vi "Acquire Spectrum.vi"(4 "Acquisition Time (s)":dbl=0.001 format="%.2p", 5 "Span (Hz)":dbl=192000.0 format="%.3p", 6 "Sample Rate (S/s)":dbl=50000000.0 format="%.2p", 7 "Reference Level":dbl format="%.2f", 8 "error in (no error)":errorcluster, 9 "RBW (Hz)":dbl=10000.0 format="%.3p", 10 "Center Frequency (Hz)":dbl=1000000000.0 format="%.6p", 11 "Instrument Handle In":refnum<k21>) -> (0 "error out":errorcluster, 2 "Spectrum":cluster{"x0":dbl, "dx":dbl, "y":sgl[]}(graph), 3 "Instrument Handle Out":refnum<k21>)   [LabVIEW 2018]
uses:
  <vilib>/RFmx/SpecAn/mx/RFmxSpecAn.llb/RFmxSpecAn Select Measurement (Single).vi
  <vilib>/RFmx/SpecAn/mx/RFmxSpecAn.llb/RFmxSpecAn Spectrum Fetch Spectrum.vi
  <vilib>/RFmx/SpecAn/mx/RFmxSpecAn.llb/RFmxSpecAn Configure IQ Power Edge Trigger.vi
panel:
  in  "Frequency Reference Source":string(combo)="OnboardClock"
  in  "Frequency (Hz)":dbl=10000000.0 format="%.6p"
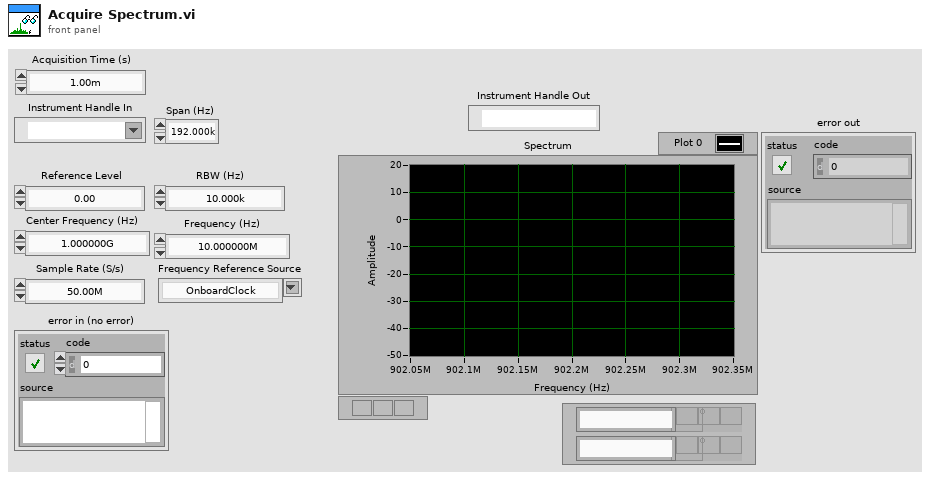
[diagram p1: front panel]
types:
  T1 = enum16{"ACP", "CCDF", "CHP", "FCnt", "Harmonics", "OBW", "SEM", "Spectrum", "Spur", "TXP", "AMPM", "DPD", "IQ", "IM", "NF", "PhaseNoise", "PAVT"}
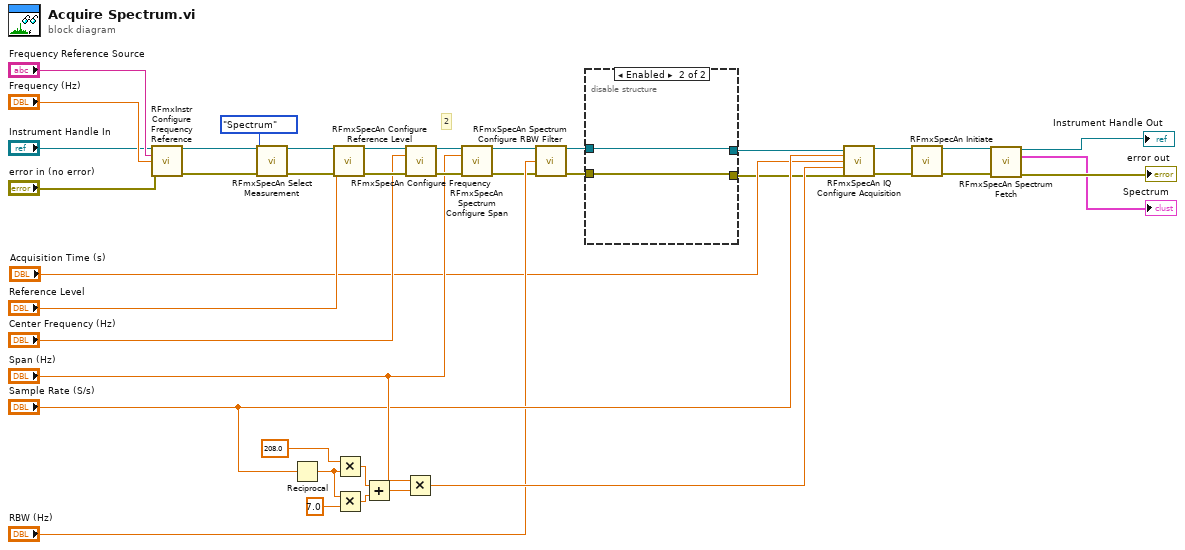
[diagram p0: block diagram]
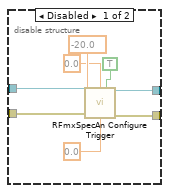
[diagram p2: hidden frame]
diagram:
  # "2"
  n1 = call <vilib>:"RFmxInstr Configure Frequency Reference.vi"("Instrument Handle In"="Instrument Handle In", "Frequency Reference Source"="Frequency Reference Source", "Frequency (Hz)"="Frequency (Hz)", "error in (no error)"="error in (no error)") -> ("Instrument Handle Out"=w16:refnum<k21>, "error out"=w15:errorcluster)  [unwired: 10 in]
  n2 = call-poly <vilib>:"RFmxSpecAn Select Measurement.vi"("Instrument Handle In"=w16, "Measurement"=T1."Spectrum", "error in (no error)"=w15) -> ("Instrument Handle Out"=w18:refnum<k21>, "error out"=w17:errorcluster)  [unwired: 11 in]
  n3 = Reciprocal(x="Sample Rate (S/s)") -> (1/x=w32:dbl)
  n4 = call <vilib>:"RFmxSpecAn Configure Reference Level.vi"("Instrument Handle In"=w18, "Reference Level"="Reference Level", "error in (no error)"=w17) -> ("Instrument Handle Out"=w37:refnum<k21>, "error out"=w36:errorcluster)  [unwired: 11 in]
  n5 = Multiply(x=208.0, y=w32) -> (x*y=w30:dbl)
  n6 = Multiply(x=w32, y=7.0) -> (x*y=w29:dbl)
  n7 = Add(x=w30, y=w29) -> (x+y=w31:dbl)
  n8 = Multiply(x="Span (Hz)", y=w31) -> (x*y=w27:dbl)
  n9 = call <vilib>:"RFmxSpecAn Configure Frequency.vi"("Instrument Handle In"=w37, "Center Frequency (Hz)"="Center Frequency (Hz)", "error in (no error)"=w36) -> ("Instrument Handle Out"=w38:refnum<k21>, "error out"=w39:errorcluster)  [unwired: 11 in]
  n10 = call <vilib>:"RFmxSpecAn Spectrum Configure Span.vi"("Instrument Handle In"=w38, "Span (Hz)"="Span (Hz)", "error in (no error)"=w39) -> ("Instrument Handle Out"=w22:refnum<k21>, "error out"=w21:errorcluster)  [unwired: 11 in]
  n11 = call <vilib>:"RFmxSpecAn Spectrum Configure RBW Filter.vi"("Instrument Handle In"=w22, "RBW (Hz)"="RBW (Hz)", "error in (no error)"=w21) -> ("Instrument Handle Out"=w3:refnum<k21>, "error out"=w4:errorcluster)  [unwired: 11 in]
  n12 = disable-structure shown="Enabled" {
    disable-tunnel: w4 -> [w46 w48]
    disable-tunnel: w3 -> [w45 w49]
    disable-tunnel: [w44 w49] -> w2
    disable-tunnel: [w43 w48] -> w1
    frame Disabled {
      n13 = call-poly <vilib>:"RFmxSpecAn Configure Trigger.vi"("Instrument Handle In"=w45, "Trigger Delay (s)"=0.0, "Enable Trigger?"=TRUE, "IQ Power Edge Level (dB or dBm)"=-20.0, "error in (no error)"=w46, "Minimum Quiet Time (s)"=0.0) -> ("Instrument Handle Out"=w44:refnum<k21>, "error out"=w43:errorcluster)  [unwired: 8 in]
    }
    frame Enabled {
    }
  }
  n14 = call <vilib>:"RFmxSpecAn IQ Configure Acquisition.vi"("Instrument Handle In"=w2, "Sample Rate (S/s)"="Sample Rate (S/s)", "Acquisition Time (s)"="Acquisition Time (s)", "Number of Records"=w27, "error in (no error)"=w1) -> ("Instrument Handle Out"=w5:refnum<k21>, "error out"=w6:errorcluster)  [unwired: 9 in]
  n15 = call <vilib>:"RFmxSpecAn Initiate.vi"("Instrument Handle In"=w5, "error in (no error)"=w6) -> ("Instrument Handle Out"=w12:refnum<k21>, "error out"=w11:errorcluster)  [unwired: 11 in, 1 out]
  n16 = call-poly <vilib>:"RFmxSpecAn Spectrum Fetch.vi"("Instrument Handle In"=w12, "error in (no error)"=w11) -> ("Instrument Handle Out"=→"Instrument Handle Out":refnum<k21>, "Spectrum"=→"Spectrum":cluster{"x0":dbl, "dx":dbl, "y":sgl[]}, "error out"=→"error out":errorcluster)  [unwired: 11 in]
